vi "ParseSendData.vi"(8 "error in (no error)":errorcluster, 11 "body":variant) -> (0 "error out":errorcluster, 3 "data send":T1)   [LabVIEW 2017, in "ServerComm.lvlib"]
uses:
  <vilib>/addons/InsightCM/Devices/Shared/Common/ServerComm/ServerComm.lvlib
  <vilib>/addons/InsightCM/Devices/Shared/Common/ServerComm/controls/DataSendBody.ctl
  <vilib>/addons/InsightCM/MessageBus/TcpApi/controls/TcpMessageReference.ctl
  <vilib>/addons/InsightCM/Devices/Shared/Common/ServerComm/controls/DataSendMode.ctl
  <vilib>/addons/InsightCM/MessageBus/Base/controls/IRoutingSource.ctl
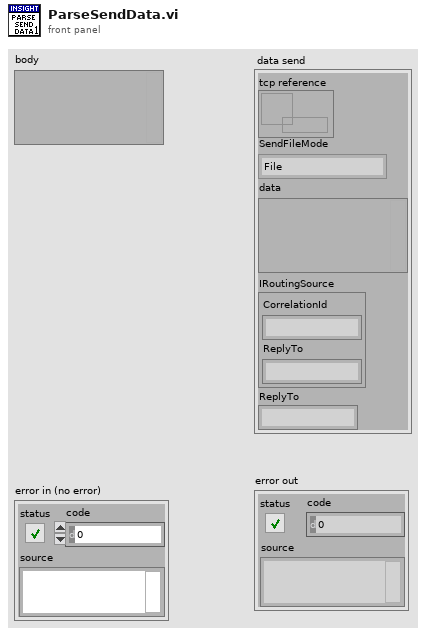
[diagram p1: front panel]
types:
  T1 = typedef "ServerComm.lvlib/DataSendBody.ctl" = cluster{"tcp reference":T2, "SendFileMode":T3, "data":variant, "IRoutingSource":T4, "ReplyTo":string}
  T2 = typedef "TcpMessageReference.ctl" = refnum<data-value>
  T3 = typedef "ServerComm.lvlib/DataSendMode.ctl" = enum16{"File", "InMemoryFile", "Stream", "StreamFileBlock", "ByteArray", "NoOp", "UnknownData"}
  T4 = typedef "IRoutingSource.ctl" = cluster{"CorrelationId":string, "ReplyTo":string}
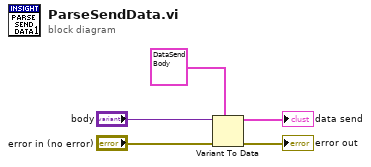
[diagram p0: block diagram]
diagram:
  n1 = Variant To Data(error in="error in (no error)", type=T1 {"tcp reference"=refnum, "SendFileMode"=enum."File", "data"=variant, "IRoutingSource"={"CorrelationId"="", "ReplyTo"=""}, "ReplyTo"=""} ("DataSend"), Variant="body") -> (data=→"data send":T1, error out=→"error out":errorcluster)
